vi "Engine-DI-InjSplits.vi"(8 "error in (no error)":errorcluster, 11 "DCM-DSI.lvclass":refnum<class "DCM-DSI.lvclass">) -> (0 "error out":errorcluster, 1 "Inj Qtys DI-B":sgl[][](array[numeric]), 2 "Inj Qtys DI-A":sgl[][](array[numeric]), 3 "DCM-DSI.lvclass":refnum<class "DCM-DSI.lvclass">)   [LabVIEW 2016, in "DSI-RT.lvlib"]
uses:
  DSI-RT.lvlib
  Classes/DCM-DSI/DCM-DSI.lvclass
  Classes/DCM-DSI/Read Channels.vi
  Classes/DCM-DSI/Write Channels.vi
  <vilib>/addons/Software Calibration Management/xSCM/FaultPoint.xnode
  <vilib>/addons/Software Calibration Management/xSCM/CalPoint.xnode
  <vilib>/addons/Software Calibration Management/xSCM/ni_scm.dll
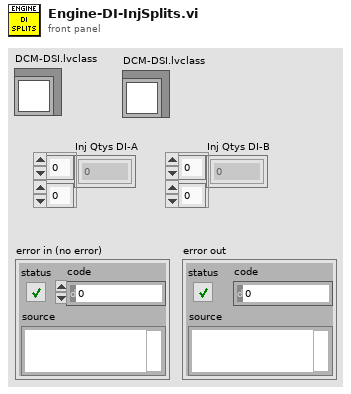
[diagram p1: front panel]
types:
  T1 = typedef "DCM-DSI.lvclass/Channel.ctl" = cluster{"Name":string, "Unit":string, "Value":sgl}
  T2 = typedef "DSI-Shared.lvlib/Engine-Channel.ctl" = cluster{"Name":string, "Unit":string, "Value":sgl}
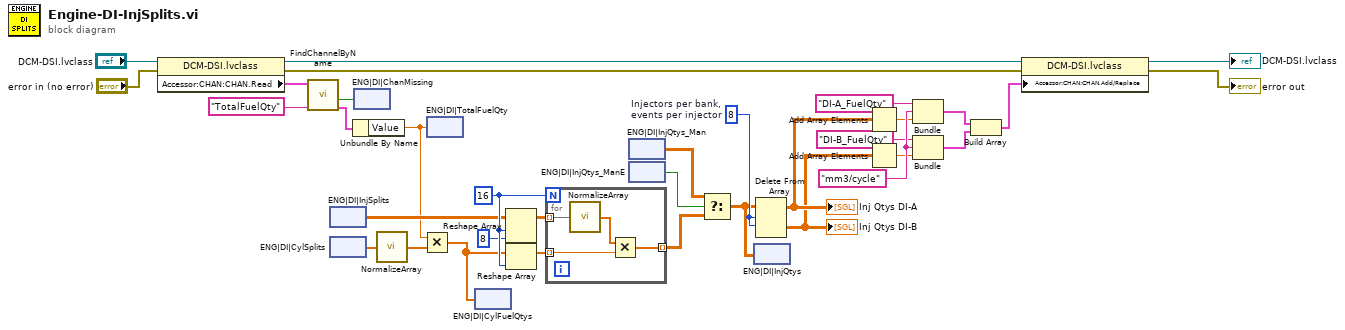
[diagram p0: block diagram]
diagram:
  w13 = "mm3/cycle"
  w16 = 8  # Injectors per bank,  events per injector
  w27 = 16
  n1 = property class="DCM-DSI.lvclass"(reference="DCM-DSI.lvclass", error in="error in (no error)") -> (reference out=w19:refnum<class "DCM-DSI.lvclass">, error out=w17:errorcluster, "Accessor:CHAN:CHAN.Read"=w18:T1[])
  n2 = call "FindChannelByName.vi"("Name"="TotalFuelQty", "CTRL.Channels in"=w18) -> ("Channel"=w29:T2, "Searching"=w30:bool)  [unwired: 6 in, 2 out]
  n3 = xnode "ENG|DI|InjSplits"() -> ("Value"=w20:sgl[][])
  n4 = xnode "ENG|DI|CylSplits"() -> ("Value"=w4:sgl[])
  n5 = Unbundle By Name(w29) -> ("Value"=w6:sgl)
  n6 = xnode "ENG|DI|ChanMissing"("Fault"=w30) -> ()
  n7 = call "NormalizeArray.vi"("Fuel Splits"=w4) -> ("Normalized Fuel Splits"=w3:sgl[])
  n8 = Multiply(x=w6, y=w3) -> (x*y=w23:sgl[])
  n9 = xnode "ENG|DI|TotalFuelQty"("Value"=w6) -> ()
  n10 = xnode "ENG|DI|CylFuelQtys"("Value"=w23) -> ()
  n11 = Reshape Array(w20, w27, 8) -> (w24:sgl[][])
  n12 = Reshape Array(w23, w27) -> (w25:sgl[])
  n13 = for {
    N: w27 -> [_]
    tunnel: w24 -> [w38] mode=indexing
    tunnel: w25 -> [w37] mode=indexing
    tunnel: [w35] -> w1 mode=indexing
    n14 = call "NormalizeArray.vi"("Fuel Splits"=w38) -> ("Normalized Fuel Splits"=w36:sgl[])
    n15 = Multiply(x=w36, y=w37) -> (x*y=w35:sgl[])
  }
  n16 = xnode "ENG|DI|InjQtys_Man"() -> ("Value"=w22:sgl[][])
  n17 = xnode "ENG|DI|InjQtys_ManE"() -> ("Value"=w21:bool)
  n18 = Select(t=w22, s=w21, f=w1) -> (s? t:f=w2:sgl[][])
  n19 = xnode "ENG|DI|InjQtys"("Value"=w2) -> ()
  n20 = Delete From Array(array=w2, length=w16, index (row)=w16) -> (deleted portion=w7:sgl[][], array with subset deleted=w8:sgl[][])  [unwired: 1 in]
  "Inj Qtys DI-A" <- w8
  "Inj Qtys DI-B" <- w7
  n21 = Add Array Elements(numeric array=w8) -> (sum=w9:sgl)
  n22 = Add Array Elements(numeric array=w7) -> (sum=w12:sgl)
  n23 = Bundle("DI-A_FuelQty", w13, "Numeric"=w9) -> (w14:cluster{string, string, "Numeric":sgl})  [unwired: 1 in]
  n24 = Bundle("DI-B_FuelQty", w13, "Numeric"=w12) -> (w15:cluster{string, string, "Numeric":sgl})  [unwired: 1 in]
  n25 = Build Array(w14, w15) -> (w5:cluster{string, string, "Numeric":sgl}[])
  n26 = property class="DCM-DSI.lvclass"(reference=w19, error in=w17, "Accessor:CHAN:CHAN.Add/Replace"=w5) -> (reference out=→"DCM-DSI.lvclass":refnum<class "DCM-DSI.lvclass">, error out=→"error out":errorcluster)
